vi "Pre_Pic_XY_Basic_BK.vi"() -> ()   [LabVIEW 2011]
panel:
  in  "TxtChoice_YScrollBar":i32(c297)
  out "TxtChoice":picture
  out "mu08TextOffsetInit":T1
  out "Vertical":i32
  out "Horizontal":i32
  out "数值":i32
  in  "Y":i32(c297)
  in  "X":i32(c297)
  out "X_Y坐标系统":picture
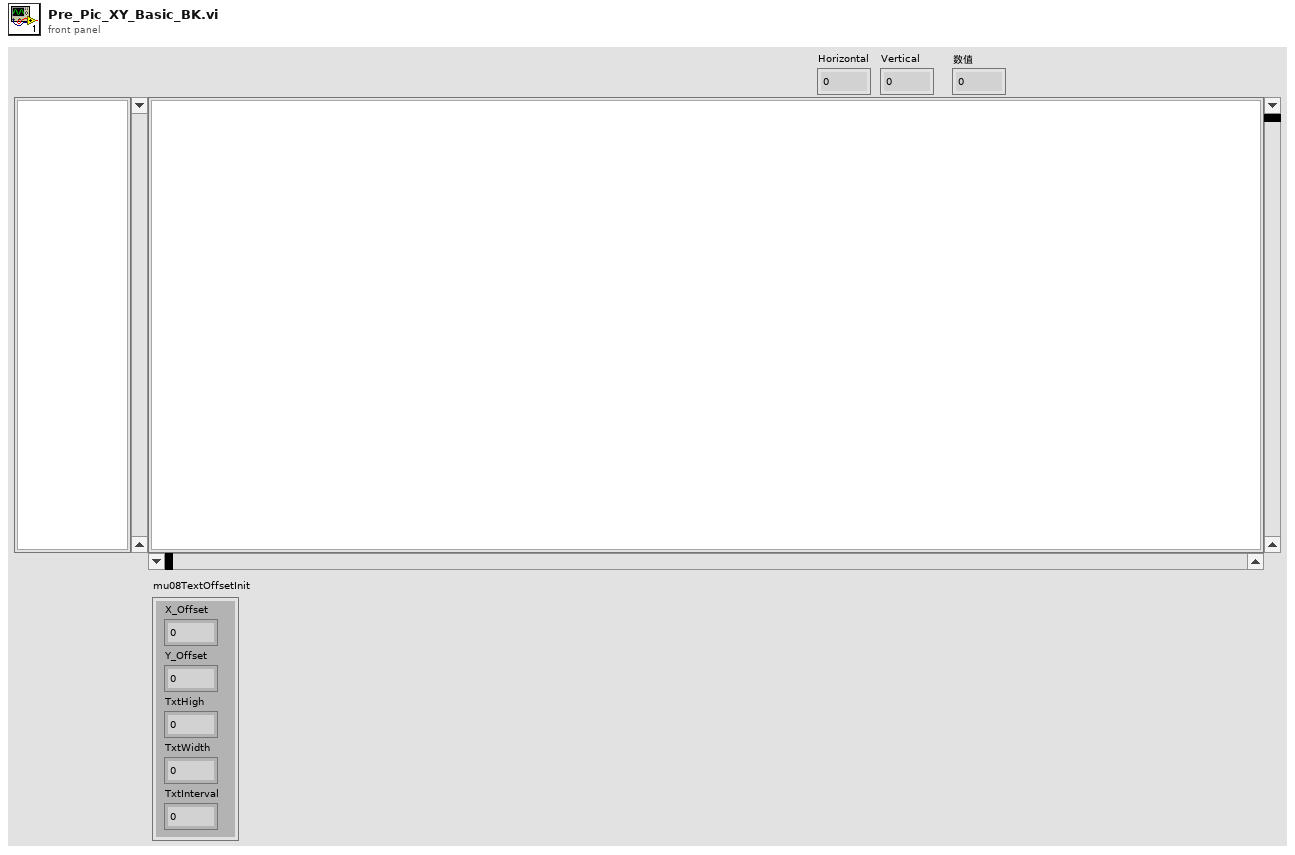
[diagram p1: front panel]
types:
  T1 = cluster{"X_Offset":u8, "Y_Offset":u8, "TxtHigh":dbl, "TxtWidth":dbl, "TxtInterval":dbl}
  T2 = typedef "LVBoundsTypeDef.ctl" = cluster{"Width":u32, "Height":u32}
  T3 = typedef "LVPoint32TypeDef.ctl" = cluster{"Horizontal":i32, "Vertical":i32}
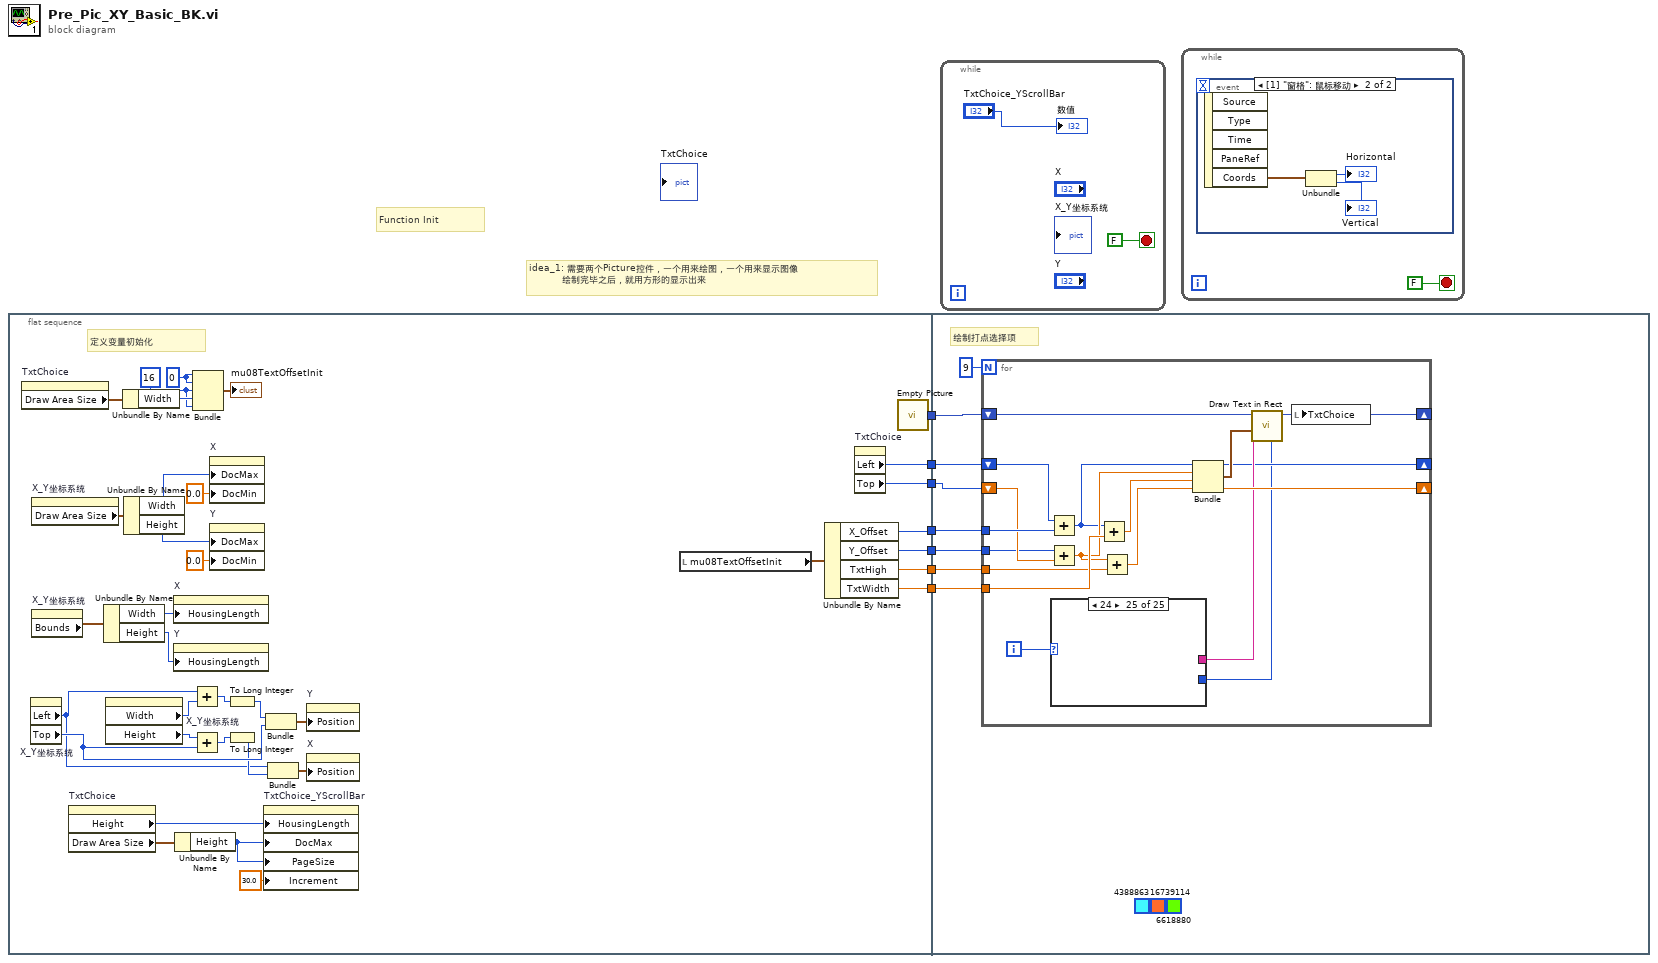
[diagram p0: block diagram]
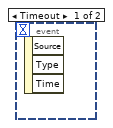
[diagram p2: hidden frame]
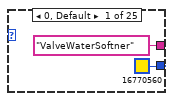
[diagram p3: hidden frame]
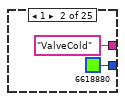
[diagram p4: hidden frame]
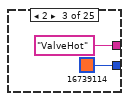
[diagram p5: hidden frame]
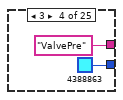
[diagram p6: hidden frame]
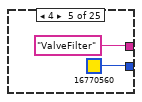
[diagram p7: hidden frame]
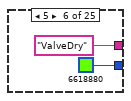
[diagram p8: hidden frame]
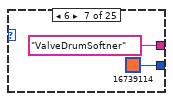
[diagram p9: hidden frame]
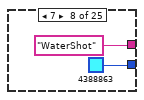
[diagram p10: hidden frame]
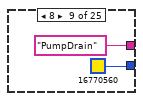
[diagram p11: hidden frame]
diagram:
  # "Function Init"
  # "idea_1: 需要两个Picture控件，一个用来绘图，一个用来显示图像\n           绘制完毕之后，就用方形的显示出来"
  n1 = flat-sequence {
    tunnel: [w20] -> w7
    tunnel: [w19] -> w6
    tunnel: [w18] -> w5
    tunnel: [w16] -> w4
    tunnel: [w15] -> w3
    tunnel: [w14] -> w2
    tunnel: [w13] -> w1
    tunnel: w7 -> [w50]
    tunnel: w6 -> [w48]
    tunnel: w5 -> [w47]
    tunnel: w4 -> [w49]
    tunnel: w3 -> [w44]
    tunnel: w2 -> [w46]
    tunnel: w1 -> [w45]
    frame #0 {
      w8 = 0
      w10 = 16
      # "定义变量初始化"
      n2 = property on="TxtChoice" class="Pict"() -> ("Draw Area Size"=w12:T2)  [unwired: 2 in, 2 out]
      n3 = property on="X_Y坐标系统" class="Pict"() -> ("Left"=w28:i32, "Top"=w30:i32)  [unwired: 2 in, 2 out]
      n4 = property on="X_Y坐标系统" class="Pict"() -> ("Draw Area Size"=w42:T2)  [unwired: 2 in, 2 out]
      n5 = property on="X_Y坐标系统" class="Pict"() -> ("Bounds"=w37:T2)  [unwired: 2 in, 2 out]
      n6 = property on="TxtChoice" class="Pict"() -> ("Height"=w24:u32, "Draw Area Size"=w23:T2)  [unwired: 2 in, 2 out]
      n7 = Unbundle By Name(w37) -> ("Width"=w36:u32, "Height"=w35:u32)
      n8 = property on="X_Y坐标系统" class="Pict"() -> ("Width"=w34:u32, "Height"=w33:u32)  [unwired: 2 in, 2 out]
      n9 = Unbundle By Name(w12) -> ("Width"=w11:u32)
      n10 = Unbundle By Name(w42) -> ("Width"=w40:u32, "Height"=w41:u32)
      n11 = property on="X" class="Scroll (严格)"("HousingLength"=w36) -> ()  [unwired: 2 in, 2 out]
      n12 = property on="Y" class="Scroll (严格)"("HousingLength"=w35) -> ()  [unwired: 2 in, 2 out]
      n13 = Unbundle By Name(w23) -> ("Height"=w21:u32)
      n14 = Add(x=w28, y=w34) -> (x+y=w26:u32)
      n15 = Add(x=w33, y=w30) -> (x+y=w25:u32)
      n16 = Bundle(w8, w8, w10, "Width"=w11, w10) -> (→"mu08TextOffsetInit":cluster{i32, i32, i32, "Width":u32, i32})  [unwired: 1 in]
      n17 = property on="X" class="Scroll (严格)"("DocMax"=w40, "DocMin"=0.0 ("滚动范围最小值")) -> ()  [unwired: 2 in, 2 out]
      n18 = property on="Y" class="Scroll (严格)"("DocMax"=w41, "DocMin"=0.0 ("滚动范围最小值")) -> ()  [unwired: 2 in, 2 out]
      n19 = To Long Integer(number=w26) -> (32bit integer=w32:i32)
      n20 = To Long Integer(number=w25) -> (32bit integer=w29:i32)
      n21 = property on="TxtChoice_YScrollBar" class="Scroll (严格)"("HousingLength"=w24, "DocMax"=w21, "PageSize"=w21, "Increment"=30.0 ("增量")) -> ()  [unwired: 2 in, 2 out]
      n22 = Bundle(w32, "Top"=w30) -> (w31:cluster{i32, "Top":i32})  [unwired: 1 in]
      n23 = Bundle("Left"=w28, w29) -> (w27:cluster{"Left":i32, i32})  [unwired: 1 in]
      n24 = property on="Y" class="Scroll (严格)"("Position"=w31) -> ()  [unwired: 2 in, 2 out]
      n25 = property on="X" class="Scroll (严格)"("Position"=w27) -> ()  [unwired: 2 in, 2 out]
      n26 = local read "mu08TextOffsetInit"() -> (w17:T1)
      n27 = Unbundle By Name(w17) -> ("X_Offset"=w16:u8, "Y_Offset"=w15:u8, "TxtHigh"=w13:dbl, "TxtWidth"=w14:dbl)
      n28 = property on="TxtChoice" class="Pict"() -> ("Left"=w19:i16, "Top"=w18:i16)  [unwired: 2 in, 2 out]
      n29 = call "Empty Picture"() -> ("empty picture"=w20:picture)
    }
    frame #1 {
      (unwired) u32 6618880 ("BG color(transparent)")
      (unwired) u32 16739114 ("BG color(transparent)")
      (unwired) u32 4388863 ("BG color(transparent)")
      # "绘制打点选择项"
      n30 = for {
        N: 9 -> [_]
        tunnel: w49 -> [w65]
        tunnel: w46 -> [w62]
        tunnel: w45 -> [w60]
        tunnel: w44 -> [w58]
        shift-right: [w57] -> _
        shift-left: w50 -> [w66]
        shift-right: [w52] -> _
        shift-left: w48 -> [w64]
        shift-right: [w55] -> _
        shift-left: w47 -> [w63]
        i -> [w54]
        n31 = Add(x=w64, y=w65) -> (x+y=w52:i16)
        n32 = Add(x=w58, y=w63) -> (x+y=w56:dbl)
        n33 = case shown="24" w54 {
          tunnel: ["ValveWaterSoftner" ("text") "ValveCold" ("text") "ValveHot" ("text") "ValvePre" ("text") "ValveFilter" ("text") "ValveDry" ("text") "ValveDrumSoftner" ("text") "WaterShot" ("text") "PumpDrain" ("text") _ _ _ _ _ _ _ _ _ _ _ _ _ _ _ _] -> w53
          tunnel: [u32 16770560 ("BG color(transparent)") u32 6618880 ("BG color(transparent)") u32 16739114 ("BG color(transparent)") u32 4388863 ("BG color(transparent)") u32 16770560 ("BG color(transparent)") u32 6618880 ("BG color(transparent)") u32 16739114 ("BG color(transparent)") u32 4388863 ("BG color(transparent)") u32 16770560 ("BG color(transparent)") _ _ _ _ _ _ _ _ _ _ _ _ _ _ _ _] -> w51
          frame 0, Default {
          }
          frame 1 {
          }
          frame 2 {
          }
          frame 3 {
          }
          frame 4 {
          }
          frame 5 {
          }
          frame 6 {
          }
          frame 7 {
          }
          frame 8 {
          }
          frame 9 {
          }
          frame 10 {
          }
          frame 11 {
          }
          frame 12 {
          }
          frame 13 {
          }
          frame 14 {
          }
          frame 15 {
          }
          frame 16 {
          }
          frame 17 {
          }
          frame 18 {
          }
          frame 19 {
          }
          frame 20 {
          }
          frame 21 {
          }
          frame 22 {
          }
          frame 23 {
          }
          frame 24 {
          }
        }
        n34 = Add(x=w52, y=w62) -> (x+y=w61:dbl)
        n35 = Add(x=w56, y=w60) -> (x+y=w55:dbl)
        n36 = Bundle(w52, w56, w61, w55) -> (w59:cluster{i16, dbl, dbl, dbl})  [unwired: 1 in]
        n37 = call <vilib>:"Draw Text in Rect.vi"("BG color(transparent)"=w51, "text"=w53, "rect"=w59, "picture"=w66) -> ("new picture"=w57:picture)  [unwired: 7 in]
        n38 = local write "TxtChoice"(w57) -> ()
      }
    }
  }
  n39 = while {
    stop <- FALSE stop-if-true
    "数值" <- "TxtChoice_YScrollBar"
  }
  n40 = while {
    stop <- FALSE stop-if-true
    n41 = event shown="[1] \"窗格\": 鼠标移动" {
      selector: _ -> [_ _]
      dyn-events: _ -> [_ _]
      timeout: _ -> [_ _]
      event Timeout {
        n42 = event-data() -> ()  [unwired: 1 in, 3 out]
      }
      event Mouse Move {
        n43 = event-data() -> ("Coords"=w90:T3)  [unwired: 1 in, 4 out]
        n44 = Unbundle(w90) -> ("Horizontal"=→"Horizontal":i32, "Vertical"=→"Vertical":i32)
      }
    }
  }
